vi "PWM Input DAQ Engine.vi"(8 "error in":errorcluster, 10 "DAQ Engine":refnum<notifier>, 11 "Sequence Context In":refnum<k7>) -> (0 "error out":errorcluster)   [LabVIEW 2023, in "LTT_TeststandSteptypes.lvlib"]
uses:
  LTT_TeststandSteptypes.lvlib
  HardwareAbstractionLayer_LVOOP/Main/Class Ref.ctl
  HardwareAbstractionLayer_LVOOP/DMM/DMM.lvclass
  HardwareAbstractionLayer_LVOOP/Function Generator/Function Generator.lvclass
  HardwareAbstractionLayer_LVOOP/Oscilloscope/Oscilloscope.lvclass
  HardwareAbstractionLayer_LVOOP/PowerSupply/PowerSupply.lvclass
  HardwareAbstractionLayer_LVOOP/Teststand/Teststand.lvclass
  HardwareAbstractionLayer_LVOOP/Analog Output/AO/AO.lvclass
  HardwareAbstractionLayer_LVOOP/Analog Input/AI/AI.lvclass
  HardwareAbstractionLayer_LVOOP/Database/Database.lvclass
  HardwareAbstractionLayer_LVOOP/Digital Output/DO_class/DO.lvclass
  HardwareAbstractionLayer_LVOOP/Digital Input/DI_class/DI.lvclass
  HardwareAbstractionLayer_LVOOP/PWM Output/PWM Output_class/PWM Output.lvclass
  HardwareAbstractionLayer_LVOOP/PWM Input/PWM Input_class/PWM Input.lvclass
  HardwareAbstractionLayer_LVOOP/NI Switch/NISwitch_class/NISwitch.lvclass
  HardwareAbstractionLayer_LVOOP/Modbus/Modbus_class/Modbus.lvclass
  HardwareAbstractionLayer_LVOOP/CAN/CAN Lib/CAN_class/CAN.lvclass
  HardwareAbstractionLayer_LVOOP/PWM Input/NI PWM Input_class/NI PWM Input.lvclass
  D:/eDCU LTT/VT LTT Project/Source Code/HardwareAbstractionLayer_LVOOP/PWM Input/PWM Input_class/PWM Input.lvclass
  HardwareAbstractionLayer_LVOOP/Main/Class Options.ctl
  <vilib>/Utility/error.llb/DialogType.ctl
  HardwareAbstractionLayer_LVOOP/Main/Main.lvclass
panel:
  in  "stop":bool
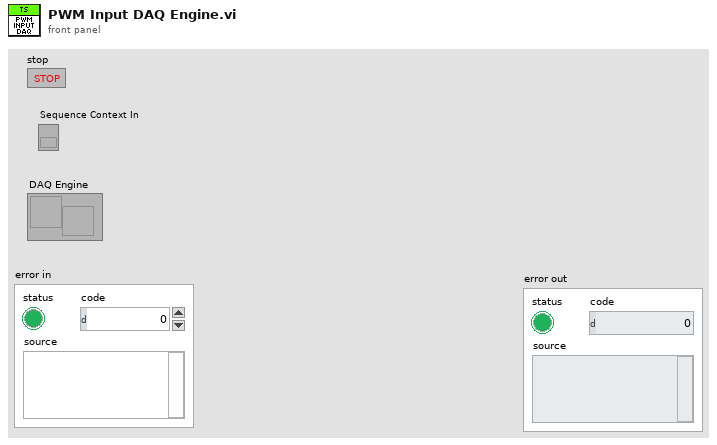
[diagram p1: front panel]
types:
  T1 = typedef "HardwareAbstractionLayer_LVOOP.lvlib/Main.lvclass/Class Ref.ctl" = cluster{"DMM":refnum<class "DMM.lvclass">, "Function Generator":refnum<class "Function Generator.lvclass">, "Oscilloscope":refnum<class "Oscilloscope.lvclass">, "PowerSupply":refnum<class "PowerSupply.lvclass">, "Teststand":refnum<class "Teststand.lvclass">, "AO":refnum<class "AO.lvclass">, "AI":refnum<class "AI.lvclass">, "Database":refnum<class "Database.lvclass">, "AO Waveform Generation":refnum<class "AO.lvclass">, "DO":refnum<class "DO.lvclass">, "DI":refnum<class "DI.lvclass">, "PWM Output":refnum<class "PWM Output.lvclass">, "PWM Input":refnum<class "PWM Input.lvclass">, "RelayOutput":refnum<class "NISwitch.lvclass">, "Modbus":refnum<class "Modbus.lvclass">, "CAN":refnum<class "CAN.lvclass">}
  T2 = typedef "HardwareAbstractionLayer_LVOOP.lvlib/Main.lvclass/Class Options.ctl" = enum16{"Init All Class", "Read All Class", "Write AI Class", "Write AO Class", "Write AO Waveform Generation", "Write DI Class", "Write DO Class", "Write PWM Input Class", "Write PWM Output Class", "Exit"}
  T3 = typedef "DialogType.ctl" = u16
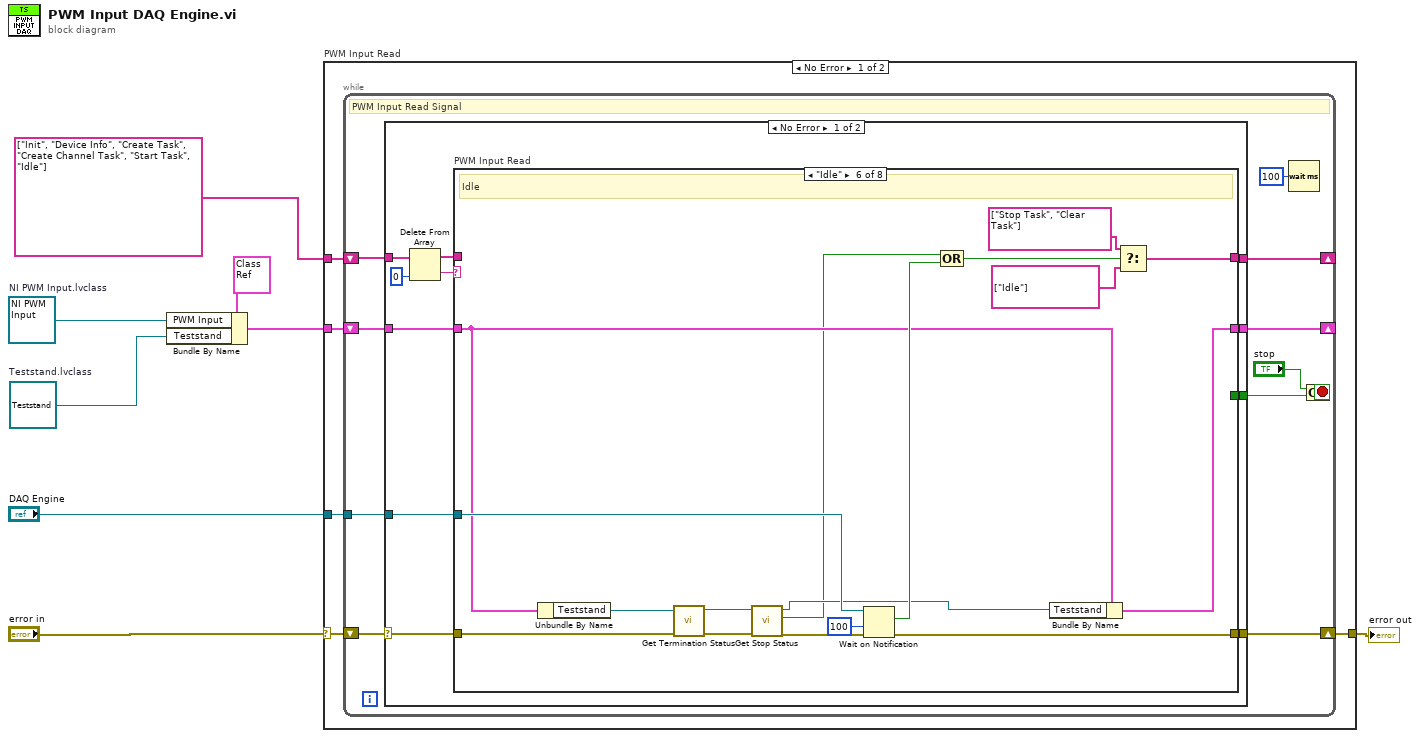
[diagram p0: block diagram]
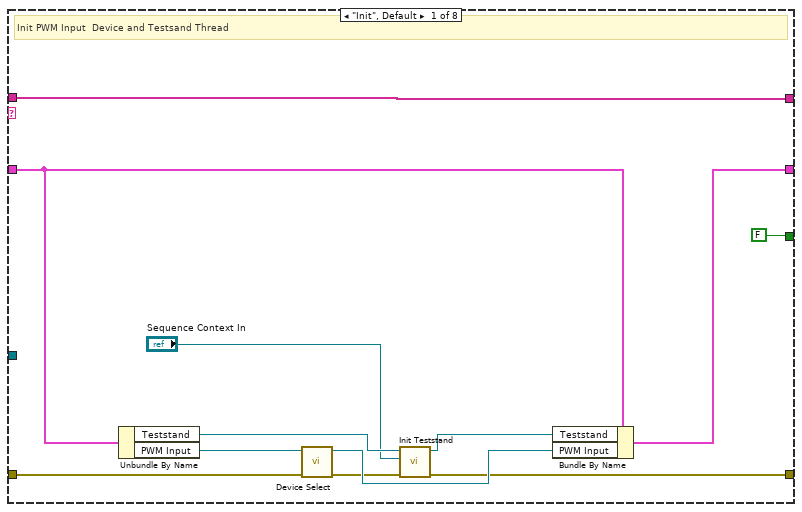
[diagram p2: hidden frame]
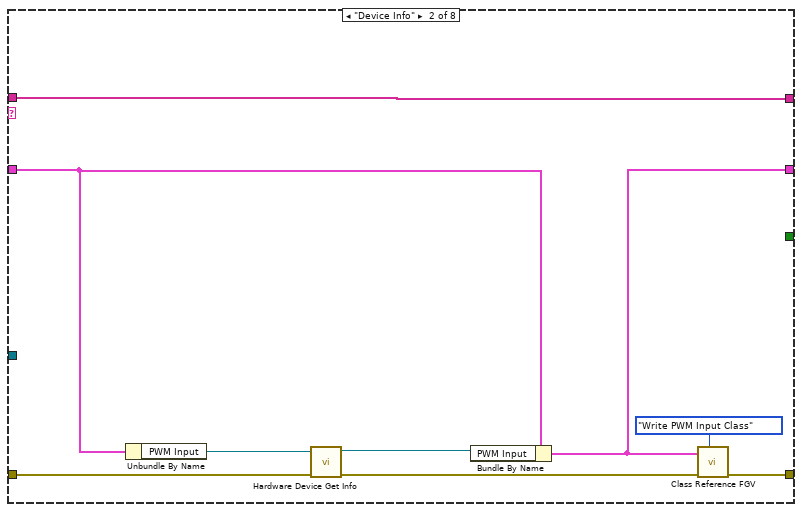
[diagram p3: hidden frame]
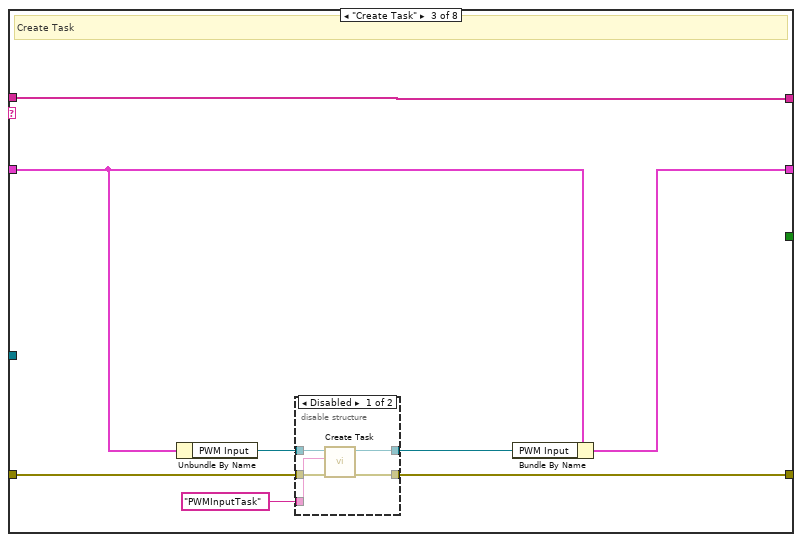
[diagram p4: hidden frame]
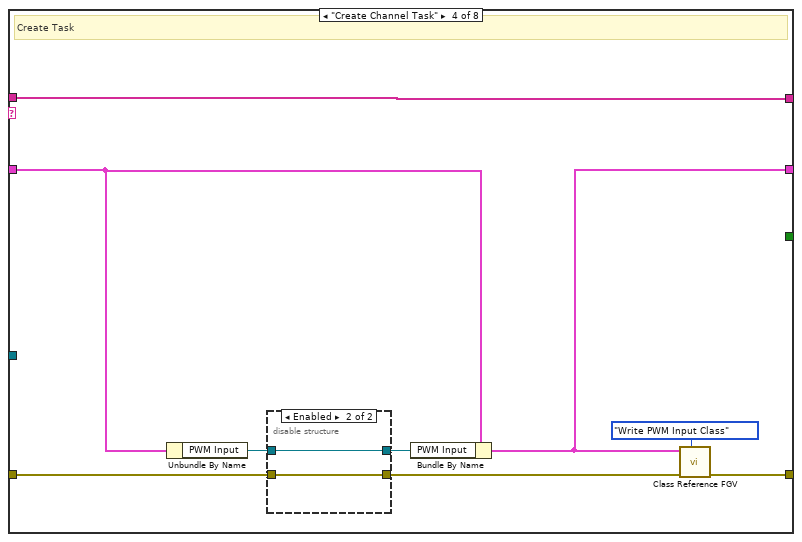
[diagram p6: hidden frame]
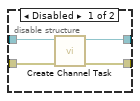
[diagram p7: hidden frame]
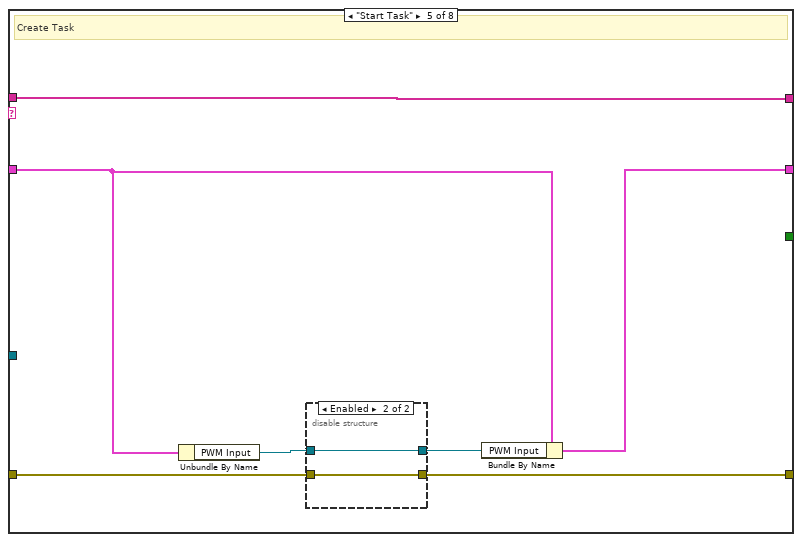
[diagram p8: hidden frame]
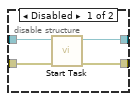
[diagram p9: hidden frame]
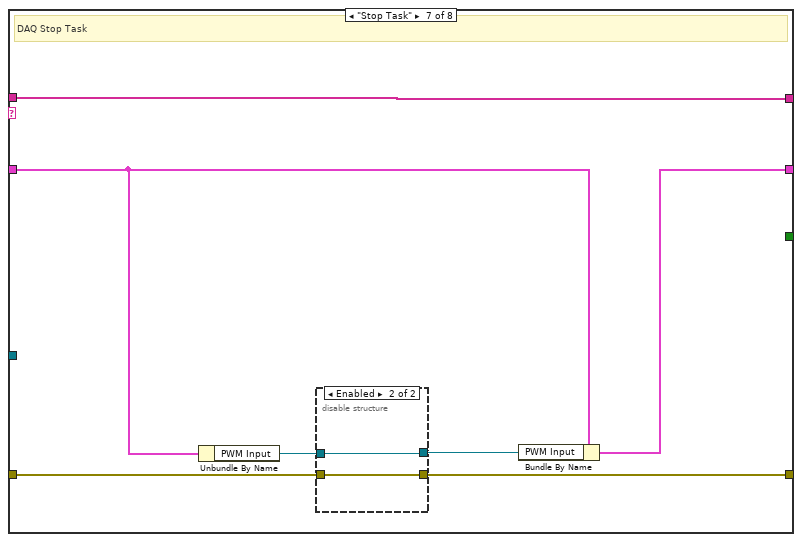
[diagram p10: hidden frame]
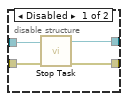
[diagram p11: hidden frame]
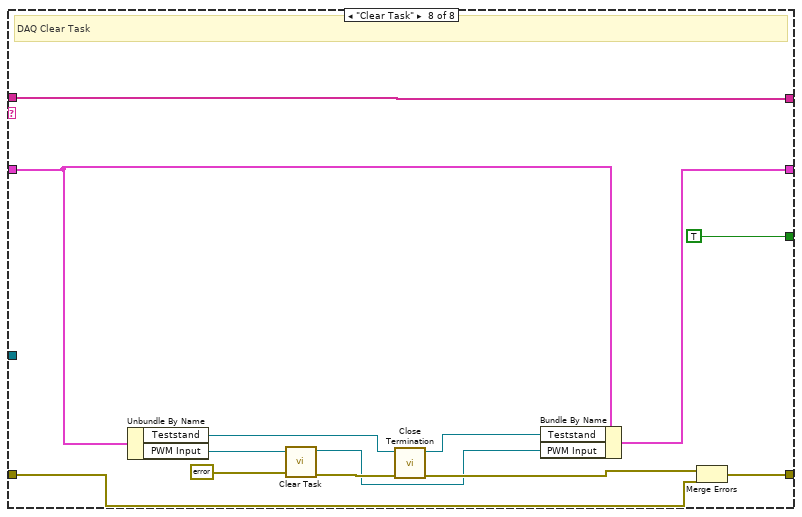
[diagram p12: hidden frame]
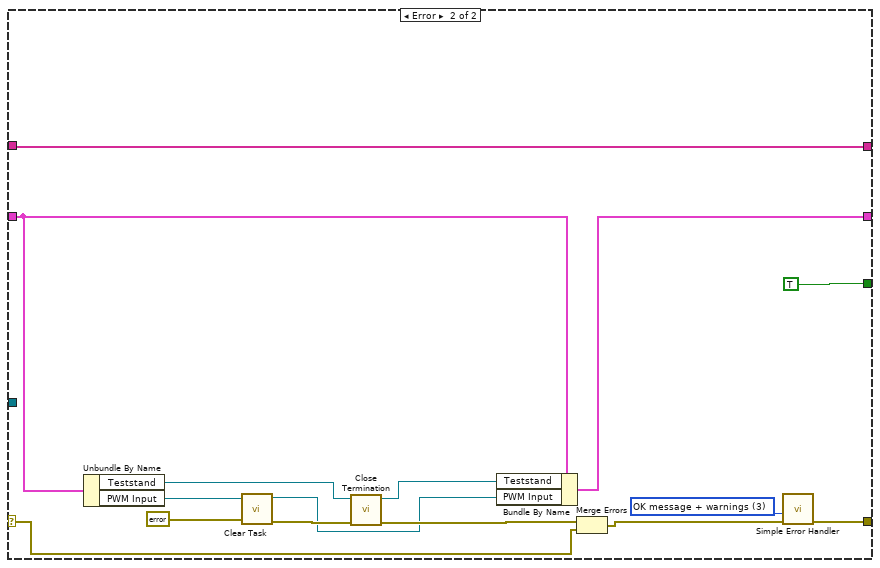
[diagram p13: hidden frame]
diagram:
  w1 = refnum<class "NI PWM Input.lvclass"> refnum  # NI PWM Input.lvclass
  w2 = refnum<class "Teststand.lvclass"> refnum  # Teststand.lvclass
  n1 = Bundle By Name(cluster=T1 {"DMM"=refnum, "Function Generator"=refnum, "Oscilloscope"=refnum, "PowerSupply"=refnum, "Teststand"=refnum, "AO"=refnum, "AI"=refnum, "Database"=refnum, "AO Waveform Generation"=refnum, "DO"=refnum, "DI"=refnum, "PWM Output"=refnum, "PWM Input"=refnum, "RelayOutput"=refnum, "Modbus"=refnum, "CAN"=refnum} ("Class Cluster"), "PWM Input"=w1, "Teststand"=w2) -> (w5:T1)
  n2 = case "PWM Input Read" shown="No Error" "error in" {
    selector: "error in" -> [w13 w158]
    tunnel: [w12 w158] -> w7
    tunnel: w5 -> [w11 _]
    tunnel: string[] ["Init", "Device Info", "Create Task", "Create Channel Task", "Start Task", "Idle"] -> [w10 _]
    tunnel: "DAQ Engine" -> [w9 _]
    frame No Error {
      n3 = while {
        shift-right: [w23] -> w12
        shift-left: w13 -> [w24]
        shift-right: [w21] -> _
        shift-left: w11 -> [w22]
        shift-right: [w19] -> _
        shift-left: w10 -> [w20]
        tunnel: w9 -> [w14]
        stop <- w16 stop-if-true
        # "PWM Input Read Signal"
        n4 = case shown="No Error" w24 {
          selector: w24 -> [w35 w147]
          tunnel: [w34 w144] -> w23
          tunnel: w22 -> [w30 w149]
          tunnel: [w29 w148] -> w21
          tunnel: w20 -> [w33 w146]
          tunnel: [w27 w146] -> w19
          tunnel: [w26 TRUE] -> w15
          tunnel: w14 -> [w25 _]
          frame No Error {
            n5 = Delete From Array(array=w33, index=0) -> (deleted portion=w32:string, array with subset deleted=w28:string[])  [unwired: 1 in]
            n6 = case "PWM Input Read" shown="\"Idle\"" w32 {
              tunnel: w35 -> [w44 w54 w59 w78 w90 w105 w120 w131]
              tunnel: [w38 w49 w58 w74 w89 w111 w119 w132] -> w34
              tunnel: w30 -> [w46 w53 w63 w79 w92 w108 w122 w141]
              tunnel: [w45 w48 w62 w73 w91 w107 w121 w140] -> w29
              tunnel: w28 -> [w47 w56 w64 w80 w93 _ w123 w142]
              tunnel: [w47 w56 w64 w80 w93 w114 w123 w142] -> w27
              tunnel: [FALSE _ _ _ _ _ _ TRUE] -> w26
              tunnel: w25 -> [_ _ _ _ _ w112 _ _]
              frame "Init", Default {
                # "Init PWM Input  Device and Testsand Thread"
                n7 = Unbundle By Name(w46) -> ("Teststand"=w40:refnum<class "Teststand.lvclass">, "PWM Input"=w41:refnum<class "PWM Input.lvclass">)
                n8 = call-dynamic "Device Select.vi"("error in (no error)"=w44, "PWM Input in"=w41) -> ("error out"=w39:errorcluster, "PWM Input out"=w43:refnum<class "PWM Input.lvclass">)  [unwired: 8 in]
                n9 = call-dynamic "Init Teststand.vi"("error in (no error)"=w39, "Sequence Context In"="Sequence Context In", "Teststand in"=w40) -> ("error out"=w38:errorcluster, "Teststand out"=w37:refnum<class "Teststand.lvclass">)  [unwired: 7 in]
                n10 = Bundle By Name(cluster=w46, "Teststand"=w37, "PWM Input"=w43) -> (w45:T1)
              }
              frame "Device Info" {
                n11 = Unbundle By Name(w53) -> ("PWM Input"=w55:refnum<class "PWM Input.lvclass">)
                n12 = call-dynamic "Hardware Device Get Info.vi"("error in (no error)"=w54, "PWM Input in"=w55) -> ("error out"=w50:errorcluster, "PWM Input out"=w52:refnum<class "PWM Input.lvclass">)  [unwired: 8 in]
                n13 = Bundle By Name(cluster=w53, "PWM Input"=w52) -> (w48:T1)
                n14 = call "Class Reference FGV.vi"("Options"=Class_Options."Write PWM Input Class", "error in"=w50, "Class Cluster In"=w48) -> ("error out"=w49:errorcluster)  [unwired: 7 in, 1 out]
              }
              frame "Create Task" {
                # "Create Task"
                n15 = Unbundle By Name(w63) -> ("PWM Input"=w61:refnum<class "PWM Input.lvclass">)
                n16 = disable-structure shown="Disabled" {
                  disable-tunnel: w61 -> [w69 w71]
                  disable-tunnel: [w68 w71] -> w60
                  disable-tunnel: w59 -> [w67 w70]
                  disable-tunnel: [w66 w70] -> w58
                  disable-tunnel: "PWMInputTask" ("Task name") -> [w65 _]
                  frame Disabled {
                    n17 = call-dynamic "Create Task.vi"("error in (no error)"=w67, "Task name"=w65, "PWM Input in"=w69) -> ("error out"=w66:errorcluster, "PWM Input out"=w68:refnum<class "PWM Input.lvclass">)  [unwired: 7 in]
                  }
                  frame Enabled {
                  }
                }
                n18 = Bundle By Name(cluster=w63, "PWM Input"=w60) -> (w62:T1)
              }
              frame "Create Channel Task" {
                # "Create Task"
                n19 = Unbundle By Name(w79) -> ("PWM Input"=w77:refnum<class "PWM Input.lvclass">)
                n20 = disable-structure shown="Enabled" {
                  disable-tunnel: w78 -> [w84 w85]
                  disable-tunnel: w77 -> [w83 w86]
                  disable-tunnel: [w82 w86] -> w76
                  disable-tunnel: [w81 w85] -> w75
                  frame Disabled {
                    n21 = call-dynamic "Create Channel Task.vi"("error in (no error)"=w84, "PWM Input in"=w83) -> ("error out"=w81:errorcluster, "PWM Input out"=w82:refnum<class "PWM Input.lvclass">)  [unwired: 8 in]
                  }
                  frame Enabled {
                  }
                }
                n22 = Bundle By Name(cluster=w79, "PWM Input"=w76) -> (w73:T1)
                n23 = call "Class Reference FGV.vi"("Options"=Class_Options."Write PWM Input Class", "error in"=w75, "Class Cluster In"=w73) -> ("error out"=w74:errorcluster)  [unwired: 7 in, 1 out]
              }
              frame "Start Task" {
                # "Create Task"
                n24 = Unbundle By Name(w92) -> ("PWM Input"=w88:refnum<class "PWM Input.lvclass">)
                n25 = disable-structure shown="Enabled" {
                  disable-tunnel: w90 -> [w97 w98]
                  disable-tunnel: [w96 w98] -> w89
                  disable-tunnel: w88 -> [w95 w99]
                  disable-tunnel: [w94 w99] -> w87
                  frame Disabled {
                    n26 = call-dynamic "Start Task.vi"("error in (no error)"=w97, "PWM Input in"=w95) -> ("error out"=w96:errorcluster, "PWM Input out"=w94:refnum<class "PWM Input.lvclass">)  [unwired: 8 in]
                  }
                  frame Enabled {
                  }
                }
                n27 = Bundle By Name(cluster=w92, "PWM Input"=w87) -> (w91:T1)
              }
              frame "Idle" {
                # "Idle"
                n28 = Unbundle By Name(w108) -> ("Teststand"=w106:refnum<class "Teststand.lvclass">)
                n29 = call-dynamic "Get Termination Status.vi"("error in (no error)"=w105, "Teststand in"=w106) -> ("error out"=w104:errorcluster, "Teststand out"=w103:refnum<class "Teststand.lvclass">)  [unwired: 7 in, 1 out]
                n30 = call-dynamic "Get Stop Status.vi"("error in (no error)"=w104, "Teststand in"=w103) -> ("error out"=w102:errorcluster, "Value"=w100:bool, "Teststand out"=w101:refnum<class "Teststand.lvclass">)  [unwired: 7 in]
                n31 = Wait on Notification(notifier=w112, timeout in ms (-1)=100, error in (no error)=w102) -> (notification=w109:bool, error out=w111:errorcluster)  [unwired: 1 in, 2 out]
                n32 = Compound Arithmetic op=OR(w100, w109) -> (w113:bool)
                n33 = Bundle By Name(cluster=w108, "Teststand"=w101) -> (w107:T1)
                n34 = Select(t=string[] ["Stop Task", "Clear Task"], s=w113, f=string[] ["Idle"]) -> (s? t:f=w114:string[])
              }
              frame "Stop Task" {
                # "DAQ Stop Task"
                n35 = Unbundle By Name(w122) -> ("PWM Input"=w118:refnum<class "PWM Input.lvclass">)
                n36 = disable-structure shown="Enabled" {
                  disable-tunnel: w120 -> [w127 w128]
                  disable-tunnel: [w126 w128] -> w119
                  disable-tunnel: w118 -> [w125 w129]
                  disable-tunnel: [w124 w129] -> w117
                  frame Disabled {
                    n37 = call-dynamic "Stop Task.vi"("error in (no error)"=w127, "PWM Input in"=w125) -> ("error out"=w126:errorcluster, "PWM Input out"=w124:refnum<class "PWM Input.lvclass">)  [unwired: 8 in]
                  }
                  frame Enabled {
                  }
                }
                n38 = Bundle By Name(cluster=w122, "PWM Input"=w117) -> (w121:T1)
              }
              frame "Clear Task" {
                # "DAQ Clear Task"
                n39 = Unbundle By Name(w141) -> ("Teststand"=w137:refnum<class "Teststand.lvclass">, "PWM Input"=w139:refnum<class "PWM Input.lvclass">)
                n40 = call-dynamic "Clear Task.vi"("error in (no error)"=errorcluster {"status"=FALSE, "code"=0, "source"=""}, "PWM Input in"=w139) -> ("error out"=w136:errorcluster, "PWM Input out"=w133:refnum<class "PWM Input.lvclass">)  [unwired: 8 in]
                n41 = call-dynamic "Close Termination.vi"("error in (no error)"=w136, "Teststand in"=w137) -> ("error out"=w135:errorcluster, "Teststand out"=w134:refnum<class "Teststand.lvclass">)  [unwired: 8 in]
                n42 = Bundle By Name(cluster=w141, "Teststand"=w134, "PWM Input"=w133) -> (w140:T1)
                n43 = Merge Errors(w135, w131) -> (w132:errorcluster)
              }
            }
          }
          frame Error {
            w143 = T3 3 items=["no dialog", "OK message", "continue or stop message", "OK message + warnings", "continue/stop + warnings"] ("type of dialog (OK msg:1)")
            n44 = Unbundle By Name(w149) -> ("Teststand"=w155:refnum<class "Teststand.lvclass">, "PWM Input"=w156:refnum<class "PWM Input.lvclass">)
            n45 = call-dynamic "Clear Task.vi"("error in (no error)"=errorcluster {"status"=FALSE, "code"=0, "source"=""}, "PWM Input in"=w156) -> ("error out"=w154:errorcluster, "PWM Input out"=w151:refnum<class "PWM Input.lvclass">)  [unwired: 8 in]
            n46 = call-dynamic "Close Termination.vi"("error in (no error)"=w154, "Teststand in"=w155) -> ("error out"=w153:errorcluster, "Teststand out"=w152:refnum<class "Teststand.lvclass">)  [unwired: 8 in]
            n47 = Bundle By Name(cluster=w149, "Teststand"=w152, "PWM Input"=w151) -> (w148:T1)
            n48 = Merge Errors(w153, w147) -> (w145:errorcluster)
            n49 = call <vilib>:"Simple Error Handler.vi"("type of dialog (OK msg:1)"=w143, "error in (no error)"=w145) -> ("error out"=w144:errorcluster)  [unwired: 3 in, 4 out]
          }
        }
        n50 = Wait (ms)(milliseconds to wait=u32 100) -> ()  [unwired: 1 out]
        n51 = Compound Arithmetic op=OR("stop", w15) -> (w16:bool)
      }
    }
    frame Error {
      # "Error"
    }
  }
  "error out" <- w7
